vi "Reset User Colors.vi"(8 "error in":errorcluster) -> (0 "error out":errorcluster)   [LabVIEW 2021, in "TSC Material Theme.lvlib" / "Material-Scheme.lvclass"]
uses:
  Material-Scheme.lvclass
  Material-Scheme.lvclass/Material-Scheme.ctl
  <resource>/dialog/lvconfig.llb/LV Config Write String.vi
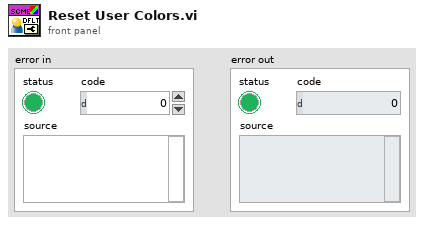
[diagram p1: front panel]
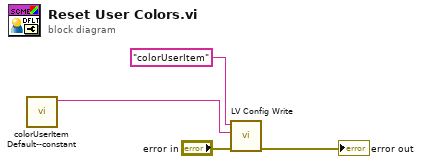
[diagram p0: block diagram]
diagram:
  n1 = call "colorUserItem Default--constant.vi"() -> ("default"=w1:string)  [unwired: 11 in]
  n2 = call-poly <resource>:"LV Config Write.vi"("error in (no error)"="error in", "value"=w1, "key"="colorUserItem") -> ("error out"=→"error out":errorcluster)  [unwired: 4 in]
